vi "create dynamic file name channel.vi"(8 "error in":errorcluster, 11 "TDMS datalogger configuration":refnum<class "TDMS datalogger configuration.lvclass">) -> (0 "error out":errorcluster, 2 "Dynamic File Channel Name":string, 3 "Dynamic File channel":refnum<class "TBM channel.lvclass">)   [LabVIEW 2018, in "TDMS datalogger configuration.lvclass"]
uses:
  TDMS datalogger configuration.lvclass
  <vilib>/NI/Tag Bus Module Framework/channel/TBM channel.lvclass
  C:/Program Files (x86)/National Instruments/LabVIEW 2018/vi.lib/NI/Tag Bus/tag/tag descriptor.lvclass
  C:/Program Files (x86)/National Instruments/LabVIEW 2018/vi.lib/NI/Configuration Framework/serializable configuration/NISE_CEF_serializable configuration.lvclass
  <vilib>/NI/Tag Bus/tag/Data Type.ctl
  <vilib>/NI/Tag Bus Module Framework/channel/channel classification.ctl
  <vilib>/NI/Configuration Framework/serializable configuration/NISE_CEF_serializable configuration.lvclass/NISE_CEF_serializable configuration.ctl
  <vilib>/Utility/LVClass/Get LV Class Name.vi
  <vilib>/NI/Configuration Framework/error generator/NISE_error generator.vi
  <vilib>/NI/Tag Bus/tag/default value polymorphs/write default value String.vi
  <vilib>/NI/Tag Bus/tag/tag descriptor.lvclass
  <vilib>/NI/Configuration Framework/serializable configuration/NISE_CEF_serializable configuration.lvclass
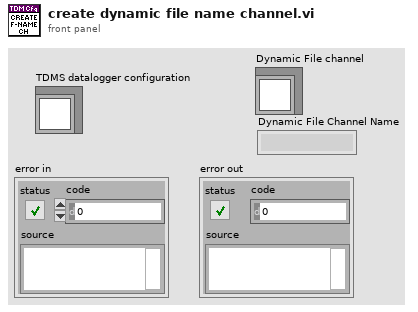
[diagram p1: front panel]
types:
  T1 = typedef "TBM channel.lvclass/channel classification.ctl" = enum16{"input data", "output data", "processing parameter", "processing result"}
  T2 = typedef "tag bus.lvlib/tag descriptor.lvclass/Data Type.ctl" = enum16{"Double", "Single", "I64", "I32", "I16", "I8", "U64", "U32", "U16", "U8", "Boolean", "String", "Array of Double", "Array of Single", "Array of I64", "Array of I32", "Array of I16", "Array of I8", "Array of U64", "Array of U32", "Array of U16", "Array of U8", "Array of Boolean", "Array of String"}
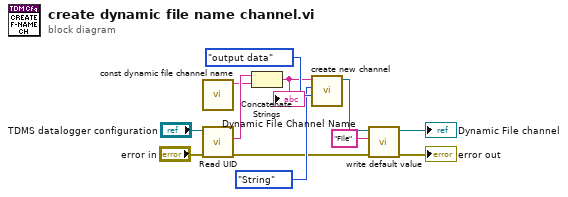
[diagram p0: block diagram]
diagram:
  n1 = call "const dynamic file channel name.vi"() -> ("enable channel"=w2:string)  [unwired: 11 in]
  n2 = call <vilib>:"Read UID.vi"("error in"="error in", "configuration in"="TDMS datalogger configuration") -> ("error out"=w6:errorcluster, "instance id"=w3:string)  [unwired: 7 in, 1 out]
  n3 = Concatenate Strings(w3, w2) -> (w4:string)
  "Dynamic File Channel Name" <- w4
  n4 = call <vilib>:"create new channel.vi"("channel classification"=channel_classification."output data", "data type"=Data_Type."String", "channel name"=w4) -> ("channel"=w10:refnum<class "TBM channel.lvclass">)  [unwired: 8 in]
  n5 = call-poly <vilib>:"write default value.vi"("error in"=w6, "default value"="File", "system tag in"=w10) -> ("error out"=→"error out":errorcluster, "system tag out"=→"Dynamic File channel":refnum<class "TBM channel.lvclass">)  [unwired: 7 in]
